vi "SetLocalSpec.vi"(8 "error in (no error)":errorcluster, 10 "Path":path, 11 "reference in":refnum<class "Test_Base.lvclass">) -> (0 "error out":errorcluster, 3 "reference in":refnum<class "Test_Base.lvclass">)   [LabVIEW 2022 SP3, in "Test_Base.lvlib" / "Test_Base.lvclass"]
uses:
  Test_Base.lvclass
  Components/TestView_Base.lvlibp/TestView_Base.lvclass
  Components/MES_Base.lvlibp/MES_Base.lvclass
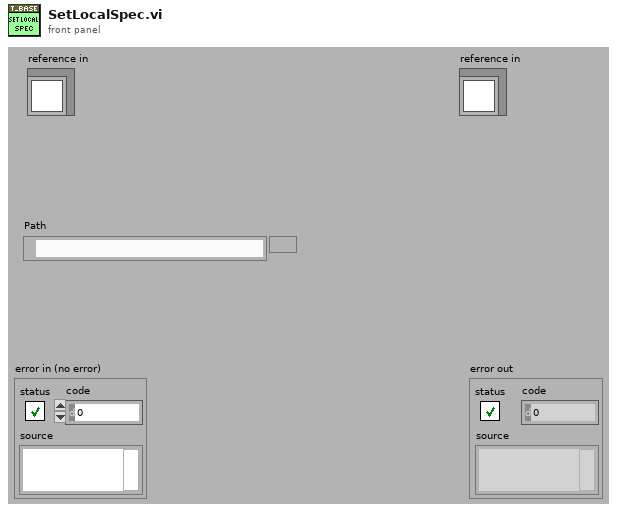
[diagram p1: front panel]
types:
  T1 = typedef "Test_Base.lvlib/Test_Base.lvclass/ObjectAttributes.ctl" = cluster{"Config":T2, "UUTIndex":i32, "Serial":string, "Batch":string, "MES":refnum<class "MES_Base.lvclass">, "TestView":refnum<class "TestView_Base.lvclass">, "LoggedIn":bool, "Abort":bool}
  T2 = typedef "Test_Base.lvlib/Test_Base.lvclass/Config.ctl" = cluster{"ContinueOnFail":bool}
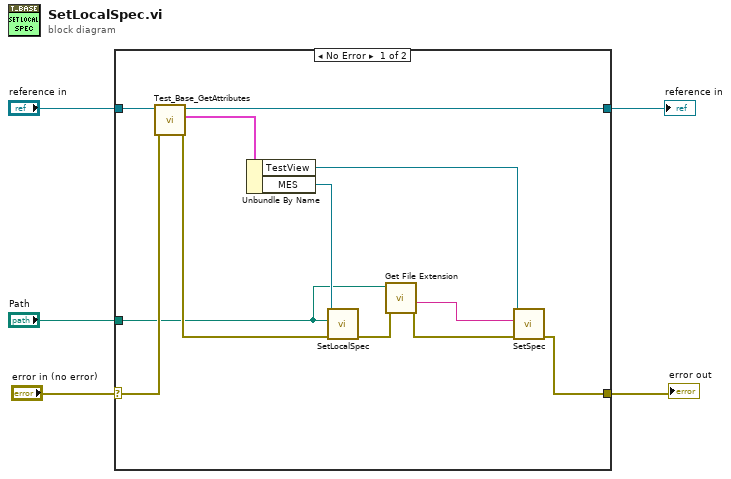
[diagram p0: block diagram]
diagram:
  n1 = case shown="No Error" "error in (no error)" {
    selector: "error in (no error)" -> [w17 w19]
    tunnel: [w11 w19] -> w4
    tunnel: [w15 w18] -> w2
    tunnel: "reference in" -> [w16 w18]
    tunnel: "Path" -> [w7 _]
    frame No Error {
      n2 = call "Test_Base_GetAttributes.vi"("error in (no error)"=w17, "reference in"=w16) -> ("error out"=w12:errorcluster, "Data"=w14:T1, "reference out"=w15:refnum<class "Test_Base.lvclass">)  [unwired: 6 in, 1 out]
      n3 = Unbundle By Name(w14) -> ("TestView"=w10:refnum<class "TestView_Base.lvclass">, "MES"=w13:refnum<class "MES_Base.lvclass">)
      n4 = call-dynamic "SetLocalSpec.vi"("error in (no error)"=w12, "Path"=w7, "reference in"=w13) -> ("error out"=w9:errorcluster)  [unwired: 7 in, 1 out]
      n5 = call <vilib>:"Get File Extension.vi"("error in (no error)"=w9, "file"=w7) -> ("error out"=w8:errorcluster, "filename without extension"=w6:string)  [unwired: 5 in, 3 out]
      n6 = call-dynamic "SetSpec.vi"("error in (no error)"=w8, "Spec"=w6, "reference in"=w10) -> ("error out"=w11:errorcluster)  [unwired: 7 in, 1 out]
    }
    frame Error {
    }
  }
  "error out" <- w4
  "reference in" <- w2
